vi "Determine Wash Cycle.vi"(8 "error in":errorcluster, 11 "Wash Options":T2) -> (0 "error out":errorcluster, 3 "Wash Cycles":T1[](array[typedef]))   [LabVIEW 8.6]
doc: "This VI uses the wash options input to build an array of states that will cycle through the appropriate wash cycles."
uses:
  Controls/State Control Enum.ctl
  Controls/Wash Options.ctl
panel:
  # "Inputs"
  # "Outputs"
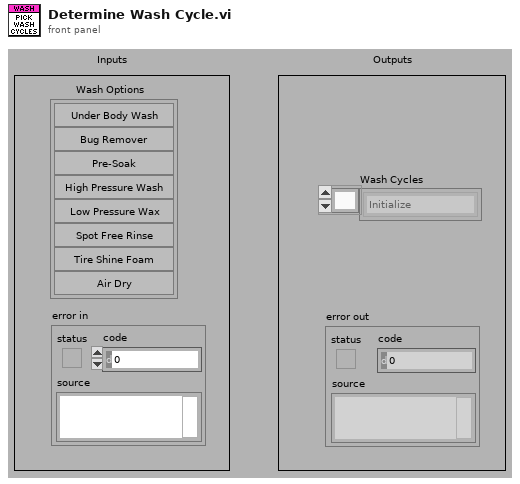
[diagram p1: front panel]
types:
  T1 = typedef "State Control Enum.ctl" = enum16{"Initialize", "Wait for Start", "Underbody Wash", "Bug Remover", "Presoak", "HP Wash", "LP Wax", "Spot Free Rinse", "Tire Shine", "Air Dry", "Exit", "Skip", "Stop"}
  T2 = typedef "Wash Options.ctl" = cluster{"Under Body Wash":bool, "Bug Remover":bool, "Pre-Soak":bool, "High Pressure Wash":bool, "Low Pressure Wax":bool, "Spot Free Rinse":bool, "Tire Shine Foam":bool, "Air Dry":bool}
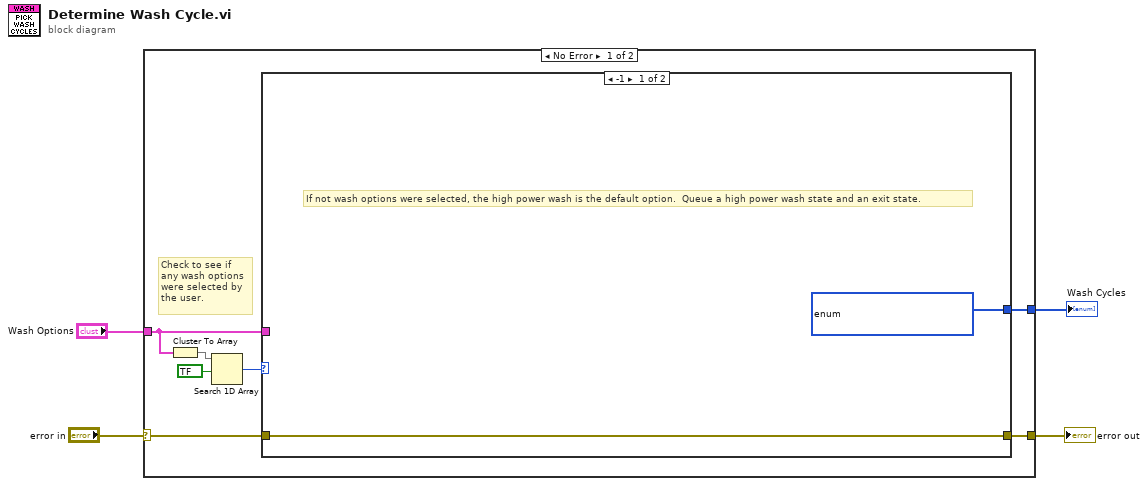
[diagram p0: block diagram]
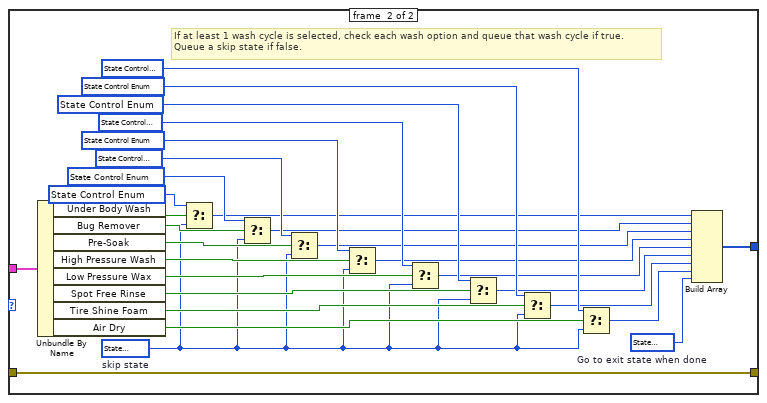
[diagram p2: hidden frame]
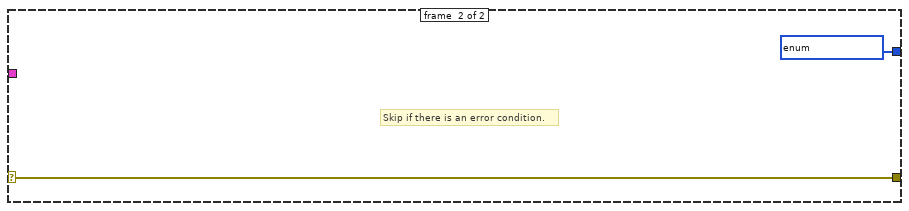
[diagram p3: hidden frame]
diagram:
  n1 = case shown="No Error" "error in" {
    selector: "error in" -> [w6 w44]
    tunnel: "Wash Options" -> [w11 _]
    tunnel: [w7 w43] -> w3
    tunnel: [w5 w44] -> w1
    frame #0 {
      # "Check to see if any wash options were selected by the user."
      n2 = Cluster To Array(cluster=w11) -> (array=w10:bool[])
      n3 = Search 1D Array(1D array=w10, element=bool ?) -> (index of element=w8:i32)  [unwired: 1 in]
      n4 = case shown="-1" w8 {
        tunnel: w11 -> [_ w17]
        tunnel: [w13 w16] -> w7
        tunnel: w6 -> [w12 w15]
        tunnel: [w12 w15] -> w5
        frame #0 {
          w13 = T1[] ? items=["Initialize", "Wait for Start", "Underbody Wash", "Bug Remover", "Presoak", "HP Wash", "LP Wax", "Spot Free Rinse", "Tire Shine", "Air Dry", "Exit", "Skip", "Stop"]
          # "If not wash options were selected, the high power wash is the default option.  Queue a high power wash state and an exit state."
        }
        frame #1 {
          w14 = T1 ?  # Go to exit state when done
          w20 = T1 ?  # skip state
          # "If at least 1 wash cycle is selected, check each wash option and queue that wash cycle if true.\nQueue a skip state if false."
          n5 = Unbundle By Name(w17) -> ("Under Body Wash"=w42:bool, "Bug Remover"=w41:bool, "Pre-Soak"=w40:bool, "High Pressure Wash"=w39:bool, "Low Pressure Wax"=w38:bool, "Spot Free Rinse"=w37:bool, "Tire Shine Foam"=w36:bool, "Air Dry"=w35:bool)
          n6 = Select(t=T1 ? ("State Control"), s=w42, f=w20) -> (s? t:f=w26:T1)
          n7 = Select(t=T1 ? ("State Control"), s=w41, f=w20) -> (s? t:f=w25:T1)
          n8 = Select(t=T1 ? ("State Control"), s=w40, f=w20) -> (s? t:f=w24:T1)
          n9 = Select(t=T1 ? ("State Control"), s=w39, f=w20) -> (s? t:f=w23:T1)
          n10 = Select(t=T1 ? ("State Control"), s=w38, f=w20) -> (s? t:f=w22:T1)
          n11 = Select(t=T1 ? ("State Control"), s=w37, f=w20) -> (s? t:f=w21:T1)
          n12 = Select(t=T1 ? ("State Control"), s=w36, f=w20) -> (s? t:f=w19:T1)
          n13 = Select(t=T1 ? ("air dry"), s=w35, f=w20) -> (s? t:f=w18:T1)
          n14 = Build Array(w26, w25, w24, w23, w22, w21, w19, w18, w14) -> (w16:T1[])
        }
      }
    }
    frame #1 {
      w43 = T1[] ? items=["Initialize", "Wait for Start", "Underbody Wash", "Bug Remover", "Presoak", "HP Wash", "LP Wax", "Spot Free Rinse", "Tire Shine", "Air Dry", "Exit", "Skip", "Stop"]
      # "Skip if there is an error condition."
    }
  }
  "Wash Cycles" <- w3
  "error out" <- w1
